vi "Sort (multiple).vi"(8 "error in (no error)":errorcluster, 9 "Use Sort Pointers (F)":bool, 10 "Sort Pointers":i32[](array[numeric]), 11 "XY-data":cluster{"X-array":dbl[], "Y-array":dbl[]}[](array[cluster]) {"Y-array" format="%.2p"; "X-array" format="%.2p"}) -> (0 "error out":errorcluster, 2 "Sorted Pointers":i32[](array[numeric]), 3 "Sorted XY-data out":cluster{"X-array":dbl[], "Y-array":dbl[]}[](array[cluster]) {"Y-array" format="%.2p"; "X-array" format="%.2p"})   [LabVIEW 2019, in "xy_utilities.lvlib"]
doc: "Sorts the input <b>XY-data</b> according to its x array.\n\nIf <b>Use Sort Pointers</b> = <b>True</b> then sort according to <b>Sort Pointers</b>.\n\nWire data to the data input to determine the polymorphic instance to use or manually select the instance."
uses:
  xy_utilities.lvlib
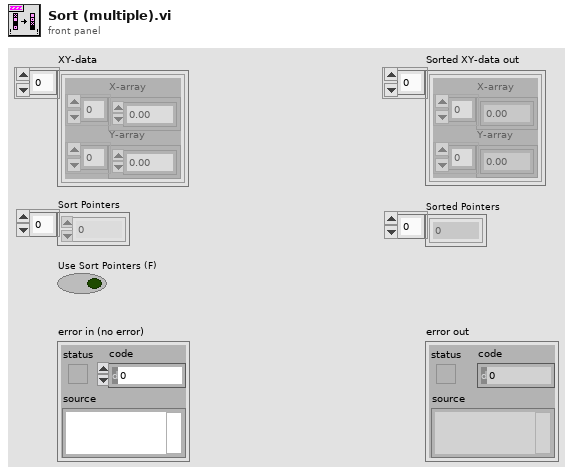
[diagram p1: front panel]
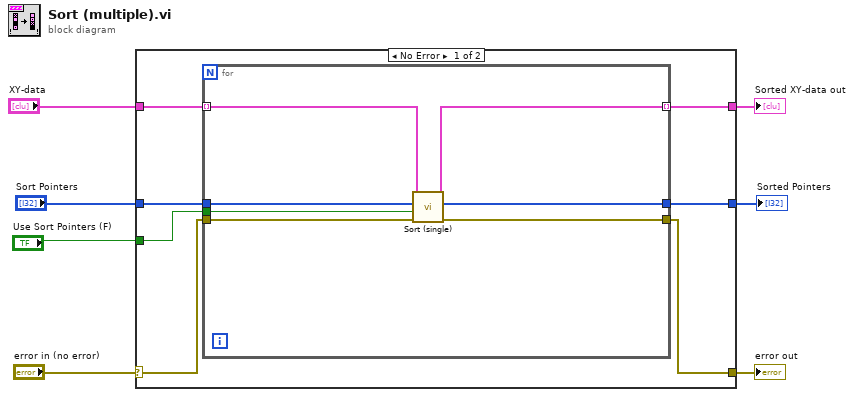
[diagram p0: block diagram]
diagram:
  n1 = case shown="No Error" "error in (no error)" {
    selector: "error in (no error)" -> [w11 w24]
    tunnel: [w12 w24] -> w6
    tunnel: "XY-data" -> [w14 w23]
    tunnel: [w13 w23] -> w4
    tunnel: [w10 w22] -> w1
    tunnel: "Use Sort Pointers (F)" -> [w9 _]
    tunnel: "Sort Pointers" -> [w8 w22]
    frame No Error {
      n2 = for {
        tunnel: w14 -> [w21] mode=indexing
        tunnel: [w20] -> w13 mode=indexing
        tunnel: [w17] -> w10
        tunnel: w9 -> [w16]
        tunnel: w8 -> [w15]
        tunnel: w11 -> [w18]
        tunnel: [w19] -> w12
        n3 = call "Sort (single).vi"("error in (no error)"=w18, "Use Sort Pointers (F)"=w16, "Sort Pointers"=w15, "XY-data"=w21) -> ("error out"=w19:errorcluster, "Sorted Pointers"=w17:i32[], "Sorted XY-data out"=w20:cluster{"X-array":dbl[], "Y-array":dbl[]})  [unwired: 5 in]
      }
    }
    frame Error {
    }
  }
  "error out" <- w6
  "Sorted XY-data out" <- w4
  "Sorted Pointers" <- w1
